vi "Digital_Bubble_Level.vi"() -> ()   [LabVIEW 2019]
uses:
  <vilib>/Platform/TimedLoop/XDataNode/timing_clust.ctl
  <vilib>/Platform/TimedLoop/XDataNode/nitl_modes.ctl
  <vilib>/Platform/TimedLoop/XDataNode/wakeup.ctl
  <vilib>/myRIO/Instrument Drivers/Onboard Devices/Accelerometer/typedefs/Accelerometer Reference.ctl
  <vilib>/myRIO/Common/Instrument Driver Framework/Utilities/typedefs/myRIO Generic Hardware Reference.ctl
  <vilib>/myRIO/Common/Instrument Driver Framework/Utilities/typedefs/Hardware Version Enum.ctl
  <vilib>/myRIO/Common/Instrument Driver Framework/Utilities/typedefs/myRIO v1.0 Reference.ctl
  <vilib>/myRIO/Common/Instrument Driver Framework/Utilities/typedefs/Generic FPGA Reference.ctl
  <vilib>/myRIO/Common/Instrument Driver Framework/myRIO v1.0/Accelerometer/typedefs/Accelerometer Channels List.ctl
  <vilib>/myRIO/Common/Instrument Driver Framework/myRIO v1.0/Accelerometer/typedefs/Accelerometer Channels Enum.ctl
  <vilib>/userDefined/High Color/nirio_resource_hc.ctl
  <vilib>/myRIO/Instrument Drivers/Onboard IO/DIO/typedefs/DIO Reference.ctl
  <vilib>/myRIO/Common/Instrument Driver Framework/myRIO v1.0/DIO/typedefs/DIO Channels List.ctl
  <vilib>/myRIO/Common/Instrument Driver Framework/myRIO v1.0/DIO/typedefs/DIO Channels Enum.ctl
  <vilib>/myRIO/Common/Instrument Driver Framework/Utilities/vis/Is FPGA Ref Available.vi
  <vilib>/myRIO/Common/Instrument Driver Framework/myRIO v1.0/DIO/vis/myRIO v1.1 Open DIO.vi
  <vilib>/myRIO/Instrument Drivers/Onboard IO/DIO/vis/Read.vi
  <vilib>/myRIO/Common/Instrument Driver Framework/myRIO v1.0/Accelerometer/vis/myRIO v1.1 Open Accelerometer.vi
  <vilib>/myRIO/Instrument Drivers/Onboard Devices/Accelerometer/vis/Read.vi
  <vilib>/myRIO/Instrument Drivers/Onboard IO/DIO/vis/Write.vi
  <vilib>/myRIO/Common/Instrument Driver Framework/Utilities/vis/Validate Channels.vi
  <vilib>/myRIO/Common/Instrument Driver Framework/myRIO v1.0/DIO/vis/myRIO v1.0 Reserve DIO.vi
  <vilib>/myRIO/Common/Instrument Driver Framework/myRIO v1.0/Accelerometer/vis/myRIO v1.0 Reserve Accelerometer.vi
  <vilib>/myRIO/Common/Instrument Driver Framework/myRIO v1.0/Resource Manager/vis/myRIO v1.0 Reserve Channel List.vi
  <vilib>/myRIO/Common/Instrument Driver Framework/myRIO v1.0/DIO/vis/myRIO v1.0 Build MUX Configuration DIO.vi
  <vilib>/myRIO/Common/Instrument Driver Framework/myRIO v1.0/Accelerometer/vis/myRIO v1.0 Build MUX Configuration Accelerometer.vi
  <vilib>/myRIO/Common/Instrument Driver Framework/myRIO v1.0/Resource Manager/vis/myRIO v1.0 Reserve Channel.vi
  <vilib>/myRIO/Common/Instrument Driver Framework/myRIO v1.0/Resource Manager/vis/myRIO v1.0 Unreserve Channel.vi
  <vilib>/myRIO/Common/Instrument Driver Framework/myRIO v1.0/Resource Manager/vis/myRIO v1.0 Create Configuration List.vi
  <vilib>/myRIO/Common/Instrument Driver Framework/myRIO v1.0/Resource Manager/vis/myRIO v1.0 Build Mutex Name.vi
  <vilib>/Utility/VariantDataType/GetNumericInfo.vi
  <vilib>/Utility/error.llb/Error Cluster From Error Code.vi
  <vilib>/myRIO/Common/Instrument Driver Framework/myRIO v1.0/myRIO v1.1 Open.vi
  <vilib>/myRIO/Common/Instrument Driver Framework/myRIO v1.0/Accelerometer/vis/myRIO v1.0 Get Scaling Constant Accelerometer.vi
  <vilib>/myRIO/Common/Instrument Driver Framework/Utilities/vis/IO Manager.vi
  <vilib>/myRIO/Common/Instrument Driver Framework/Utilities/vis/Configuration Manager.vi
  <vilib>/myRIO/Common/Instrument Driver Framework/myRIO v1.0/myRIO v1.0 Close.vi
  <vilib>/myRIO/Common/Instrument Driver Framework/myRIO v1.0/Accelerometer/vis/myRIO v1.0 Read Accelerometer.vi
  <vilib>/myRIO/Common/Instrument Driver Framework/myRIO v1.0/Resource Manager/vis/myRIO v1.0 Configure IO.vi
  <vilib>/myRIO/Common/Instrument Driver Framework/myRIO v1.0/DIO/vis/myRIO v1.0 Write DIO.vi
  <vilib>/myRIO/Common/Instrument Driver Framework/myRIO v1.0/DIO/vis/myRIO v1.0 Read DIO.vi
  <vilib>/platform/TimedLoop/XDataNode/XDataNode.xnode
  <vilib>/myRIO/Express VI/Onboard Devices/Accelerometer/Accelerometer Express VI.xnode
  <vilib>/myRIO/Instrument Drivers/Onboard Devices/Accelerometer/vis/myRIO Accelerometer Open.xnode
  <vilib>/myRIO/Express VI/Onboard Devices/LED/LED Express VI.xnode
  <vilib>/myRIO/Instrument Drivers/Onboard IO/DIO/vis/myRIO DIO Open.xnode
  <vilib>/myRIO/Express VI/Onboard Devices/Button/Button Express VI.xnode
  <vilib>/myRIO/Instrument Drivers/Onboard Devices/Accelerometer/Accelerometer.lvlib
  <vilib>/myRIO/Instrument Drivers/Onboard IO/DIO/DIO.lvlib
  <vilib>/Platform/TimedLoop/XDataNode/XDNodeRunTimeDep.lvlib
panel:
  out "error out":errorcluster
  out "Numeric 3":dbl
  out "Numeric 2":dbl
  out "Value_Bubble":string
  in  "stop 2":bool
  out "Numeric":dbl
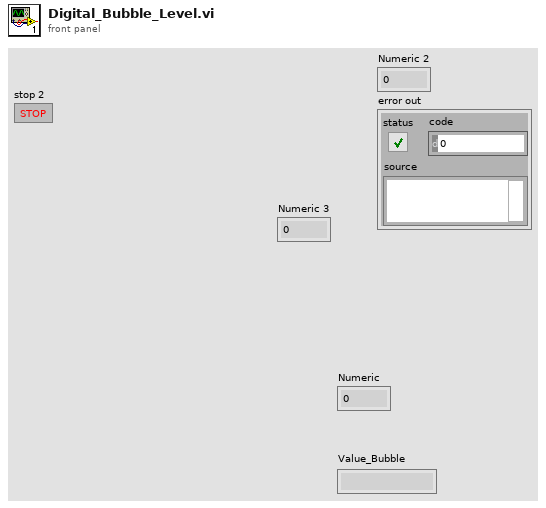
[diagram p1: front panel]
types:
  T1 = typedef "XDNodeRunTimeDep.lvlib/timing_clust.ctl" = cluster{"Expected End [f-1]":u64, "Actual End [f-1]":u64, "Finished Late? [f-1]":bool, "Expected End [i-1]":u64, "Actual End [i-1]":u64, "Finished Late? [i-1]":bool, "Expected Start [i]":u64, "Actual Start [i]":u64, "Expected Start [f]":u64, "Actual Start [f]":u64, "Source Name":string, "Structure Name":string, "Period":i64, "Deadline":i64, "Offset":i64, "Start":i64, "Priority":i32, "Timeout":i32, "Mode":T2, "Wakeup Reason":T3, "Error":errorcluster, "Source Type":string, "Secondary Source Type":string, "Global End Time":u64, "Global Start Time":u64, "Frame Duration":u64, "Iteration Duration":u64, "Assigned CPU":i32, "I/O Scan Engine Mode":u32}
  T2 = typedef "XDNodeRunTimeDep.lvlib/nitl_modes.ctl" = enum32{"No Change", "Process missed periods, maintain original phase", "Discard missed periods, maintain original phase", "Process missed periods, ignore original phase", "Discard missed periods, ignore original phase"}
  T3 = typedef "XDNodeRunTimeDep.lvlib/wakeup.ctl" = enum32{"Normal", "Aborted", "Asynchronous wakeup", "Timing source error", "Timed loop error", "Timeout"}
  T4 = enum16{"open", "replace", "create", "open or create", "replace or create", "replace or create with confirmation"}
  T5 = typedef "DIO.lvlib/DIO Reference.ctl" = cluster{"myRIO Reference":T6, "DIO Channels List":T10}
  T6 = typedef "myRIO Generic Hardware Reference.ctl" = cluster{"myRIO Model":T7, "myRIO Hardware Reference":T8}
  T7 = typedef "Hardware Version Enum.ctl" = enum16{"Unknown", "myRIO-1900", "myRIO-1950", "roboRIO", "NI ELVIS RIO CM", "ELVIS III"}
  T8 = typedef "myRIO v1.0 Reference.ctl" = cluster{"Generic FPGA Reference":T9, "Allow multiple opens":bool}
  T9 = typedef "Generic FPGA Reference.ctl" = refnum<k20>
  T10 = typedef "DIO Channels List.ctl" = T11[]
  T11 = typedef "DIO Channels Enum.ctl" = enum16{"Not Connected", "C/DIO0", "C/DIO1", "C/DIO2", "C/DIO3", "C/DIO4", "C/DIO5", "C/DIO6", "C/DIO7", "A/DIO0", "A/DIO1", "A/DIO2", "A/DIO3", "A/DIO4", "A/DIO5", "A/DIO6", "A/DIO7", "A/DIO8", "A/DIO9", "A/DIO10", "A/DIO11", "A/DIO12", "A/DIO13", "A/DIO14", "A/DIO15", "A/DIO16", "A/DIO17", "A/DIO18", "A/DIO19", "B/DIO0", "B/DIO1", "B/DIO2", "B/DIO3", "B/DIO4", "B/DIO5", "B/DIO6", "B/DIO7", "B/DIO8", "B/DIO9", "B/DIO10", "B/DIO11", "B/DIO12", "B/DIO13", "B/DIO14", "B/DIO15", "B/DIO16", "B/DIO17", "B/DIO18", "B/DIO19", "LED0", "LED1", "LED2", "LED3", "Button0", "DIO/DIO0", "DIO/DIO1", "DIO/DIO2", "DIO/DIO3", "DIO/DIO4", "DIO/DIO5", "DIO/DIO6", "DIO/DIO7", "DIO/DIO8", "DIO/DIO9", "SPI/CS0", "SPI/CS1", "SPI/CS2", "SPI/CS3", "LED RADIO (Green)", "LED RADIO (Red)", "LED COMM (Green)", "LED COMM (Red)", "LED MODE (Green)", "LED MODE (Red)"}
  T12 = typedef "nirio_resource_hc.ctl" = tag
  T13 = typedef "Accelerometer.lvlib/Accelerometer Reference.ctl" = cluster{"myRIO Reference":T6, "Accelerometer Channels List":T14, "LSB Weight":dbl}
  T14 = typedef "Accelerometer Channels List.ctl" = T15[]
  T15 = typedef "Accelerometer Channels Enum.ctl" = enum16{"Not Connected", "X-Axis", "Y-Axis", "Z-Axis"}
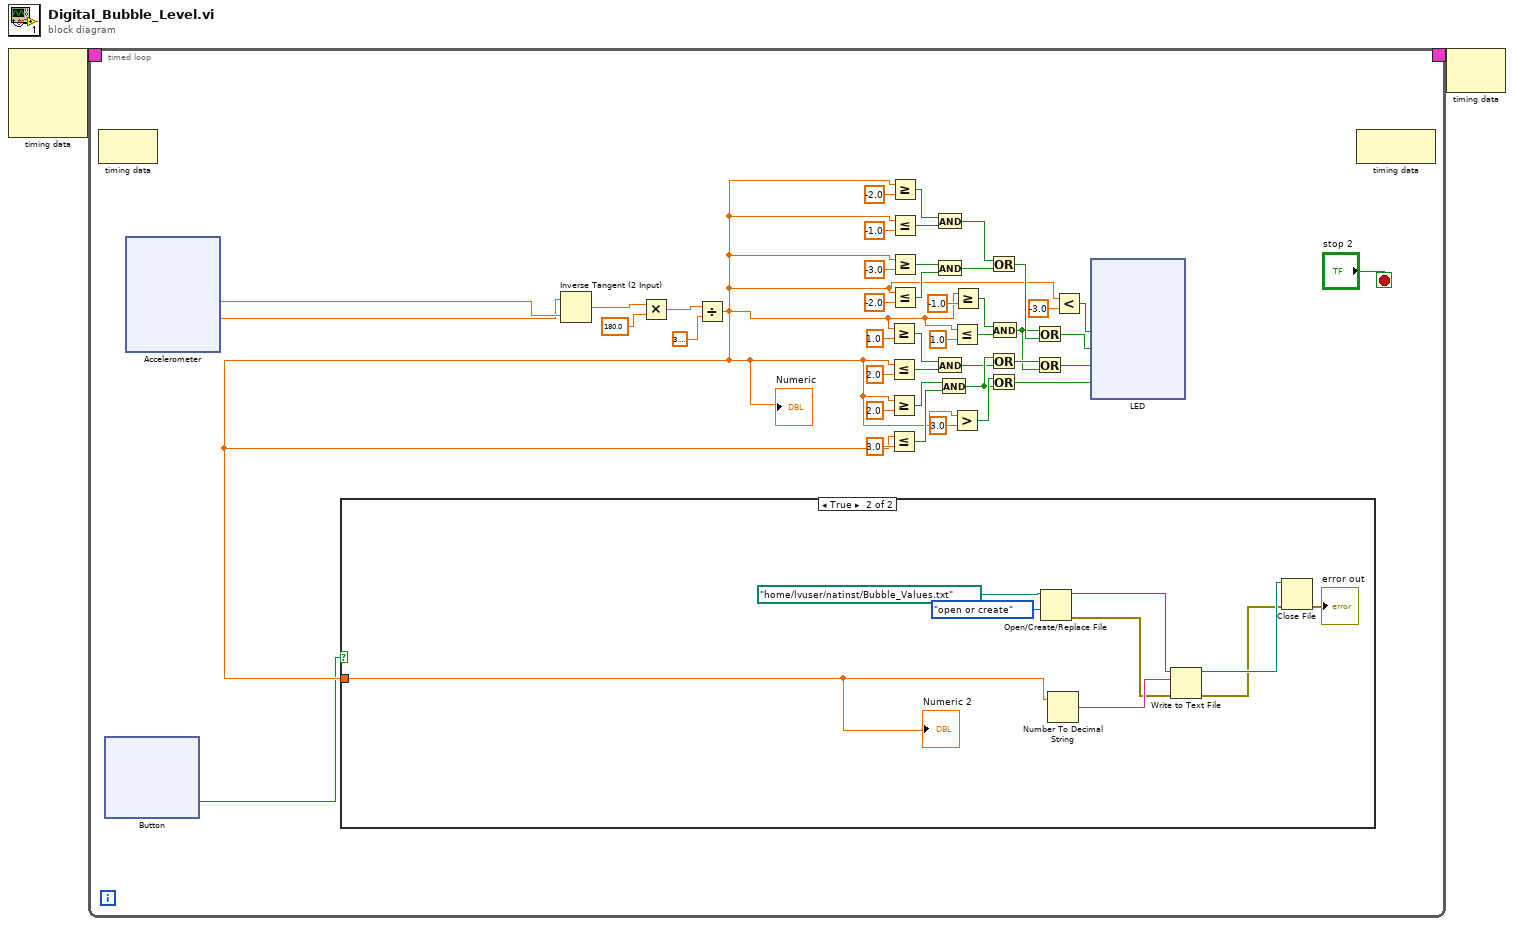
[diagram p0: block diagram]
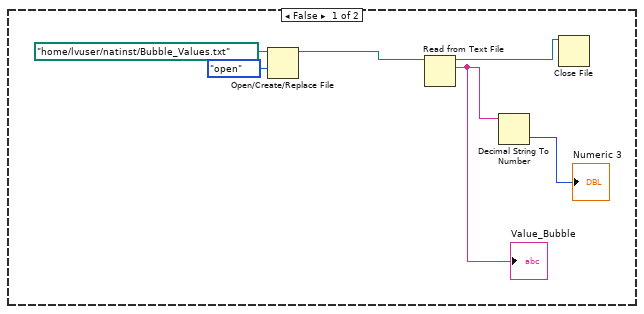
[diagram p2: hidden frame]
diagram:
  n1 = node-c288() -> (w2:T1)  [unwired: 4 in]
  n2 = timed-loop {
    timing: w2 -> [_]
    timing-out: [_] -> w1
    stop <- "stop 2" stop-if-true
    n3 = node-c288() -> ()  [unwired: 1 in, 1 out]
    n4 = xnode "Button"() -> ("Value"=w3:bool)  [unwired: 1 in, 1 out]
    n5 = xnode "Accelerometer"() -> ("X-Axis"=w45:dbl, "Y-Axis"=w44:dbl)  [unwired: 1 in, 2 out]
    n6 = Inverse Tangent (2 Input)(1:w45, 2:w44) -> (0:w43:dbl)
    n7 = Multiply(x=w43, y=180.0) -> (x*y=w41:dbl)
    n8 = Divide(x=w41, y=3.141592653589793) -> (x/y=w4:dbl)
    "Numeric" <- w4
    n9 = case shown="True" w3 {
      tunnel: w4 -> [_ w59]
      frame False {
        n10 = Open/Create/Replace File(file path (use dialog)=path "/home/lvuser/natinst/Bubble_Values.txt", operation (0:open)=T4."open") -> (refnum out=w50:refnum<file>)  [unwired: 4 in, 2 out]
        n11 = Read from Text File(file (use dialog)=w50) -> (refnum out=w49:refnum<file>, text=w47:string)  [unwired: 3 in, 2 out]
        "Value_Bubble" <- w47
        n12 = Decimal String To Number(string=w47) -> (number=→"Numeric 3":i32)  [unwired: 2 in, 1 out]
        n13 = Close File(refnum=w49) -> ()  [unwired: 1 in, 2 out]
      }
      frame True {
        n14 = Open/Create/Replace File(file path (use dialog)=path "/home/lvuser/natinst/Bubble_Values.txt", operation (0:open)=T4."open or create") -> (refnum out=w56:refnum<file>, error out=w54:errorcluster)  [unwired: 4 in, 1 out]
        n15 = Number To Decimal String(number=w59) -> (decimal integer string=w60:string)  [unwired: 1 in]
        n16 = Write to Text File(file (use dialog)=w56, text=w60, error in=w54) -> (refnum out=w58:refnum<file>, error out=w53:errorcluster)  [unwired: 1 in, 1 out]
        n17 = Close File(refnum=w58, error in=w53) -> (error out=→"error out":errorcluster)  [unwired: 1 out]
        "Numeric 2" <- w59
      }
    }
    n18 = Greater Or Equal?(x=w4, y=1.0) -> (x >= y?=w34:bool)
    n19 = Less Or Equal?(x=w4, y=2.0) -> (x <= y?=w33:bool)
    n20 = Greater Or Equal?(x=w4, y=2.0) -> (x >= y?=w38:bool)
    n21 = Less Or Equal?(x=w4, y=3.0) -> (x <= y?=w37:bool)
    n22 = Greater Or Equal?(x=w4, y=-2.0) -> (x >= y?=w26:bool)
    n23 = Less Or Equal?(x=w4, y=-1.0) -> (x <= y?=w25:bool)
    n24 = Greater Or Equal?(x=w4, y=-3.0) -> (x >= y?=w22:bool)
    n25 = Less Or Equal?(x=w4, y=-2.0) -> (x <= y?=w21:bool)
    n26 = And(x=w26, y=w25) -> (x .and. y?=w11:bool)
    n27 = And(x=w22, y=w21) -> (x .and. y?=w10:bool)
    n28 = And(x=w34, y=w33) -> (x .and. y?=w14:bool)
    n29 = And(x=w38, y=w37) -> (x .and. y?=w15:bool)
    n30 = Less Or Equal?(x=w4, y=1.0) -> (x <= y?=w30:bool)
    n31 = Greater?(x=w4, y=3.0) -> (0:w17:bool)
    n32 = Greater Or Equal?(x=w4, y=-1.0) -> (x >= y?=w29:bool)
    n33 = Or(x=w11, y=w10) -> (x .or. y?=w8:bool)
    n34 = Or(x=w15, y=w14) -> (x .or. y?=w13:bool)
    n35 = Or(x=w17, y=w15) -> (x .or. y?=w16:bool)
    n36 = And(x=w29, y=w30) -> (x .and. y?=w7:bool)
    n37 = Or(x=w7, y=w8) -> (x .or. y?=w6:bool)
    n38 = Or(x=w13, y=w7) -> (x .or. y?=w12:bool)
    n39 = Less?(x=w4, y=-3.0) -> (x < y?=w9:bool)
    n40 = xnode "LED"("LED0"=w9, "LED1"=w6, "LED2"=w12, "LED3"=w16) -> ()  [unwired: 1 in, 1 out]
    n41 = node-c288() -> ()  [unwired: 1 in, 1 out]
  }
  n42 = node-c288(w1) -> ()  [unwired: 1 out]
